vi "_create_uuts_and_aliases.vi"(8 "error in":errorcluster) -> (0 "error out":errorcluster, 4 "log":string)   [LabVIEW 2024]
uses:
  <vilib>/Plug-In SDKs/Clients/Metadata/UUT.ctl
  <vilib>/Plug-In SDKs/Clients/Metadata/Extension.ctl
  <vilib>/Plug-In SDKs/Clients/Metadata Store V1/Metadata Store Client.lvlibp/API/Metadata Store V1/Create UUT.vi
  <vilib>/Plug-In SDKs/Clients/Metadata Store V1/Metadata Store Client.lvlibp/API/Metadata Store V1/Create Alias (Metadata - UUT).vi
  <vilib>/Plug-In SDKs/Clients/Metadata Store V1/Metadata Store Client.lvlibp
  <vilib>/Plug-In SDKs/Clients/Metadata/NI Metadata Types.lvlib
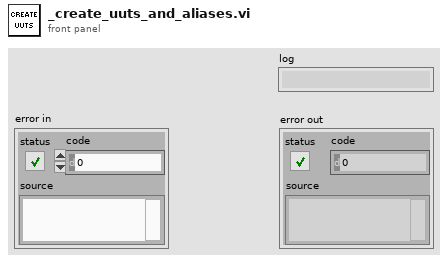
[diagram p1: front panel]
types:
  T1 = typedef "NI Metadata Types.lvlib/UUT.ctl" = cluster{"model name":string, "family":string, "manufacturers":string[], "part number":string, "id":string, "link":string, "extensions":T2[], "schema id":string}
  T2 = typedef "NI Metadata Types.lvlib/Extension.ctl" = cluster{"name":string, "value":string}
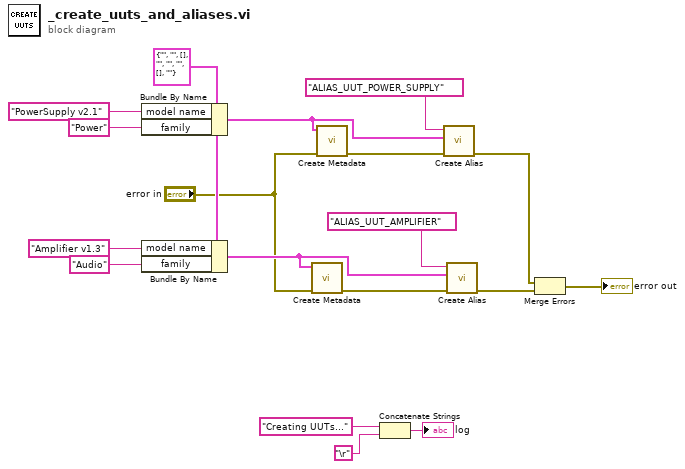
[diagram p0: block diagram]
diagram:
  w6 = T1 {"model name"="", "family"="", "manufacturers"=[], "part number"="", "id"="", "link"="", "extensions"=[], "schema id"=""} ("uut")
  n1 = Bundle By Name(cluster=w6, "model name"="PowerSupply v2.1" ("operator name"), "family"="Power" ("operator name")) -> (w12:T1)
  n2 = Bundle By Name(cluster=w6, "model name"="Amplifier v1.3" ("serial number"), "family"="Audio" ("model")) -> (w15:T1)
  n3 = call-poly <vilib>:"Create Metadata.vi"("error in"="error in", "uut"=w15) -> ("error out"=w10:errorcluster)  [unwired: 8 in, 1 out]
  n4 = call-poly <vilib>:"Create Metadata.vi"("error in"="error in", "uut"=w12) -> ("error out"=w11:errorcluster)  [unwired: 8 in, 1 out]
  n5 = Concatenate Strings("Creating UUTs..." ("role"), "\r") -> (→"log":string)
  n6 = call-poly <vilib>:"Create Alias.vi"("error in"=w11, "uut"=w12, "alias name"="ALIAS_UUT_POWER_SUPPLY") -> ("error out"=w16:errorcluster)  [unwired: 7 in, 1 out]
  n7 = call-poly <vilib>:"Create Alias.vi"("error in"=w10, "uut"=w15, "alias name"="ALIAS_UUT_AMPLIFIER") -> ("error out"=w17:errorcluster)  [unwired: 7 in, 1 out]
  n8 = Merge Errors(w16, w17) -> (→"error out":errorcluster)
